vi "Measure.vi"(8 "error in (no error)":errorcluster, 11 "Measurement2D in":refnum<class "Measurement2D.lvclass">) -> (0 "error out":errorcluster, 1 "Current Value":dbl, 2 "Result":dbl, 3 "Measurement2D out":refnum<class "Measurement2D.lvclass">)   [LabVIEW 2014, in "Measurement2D.lvclass"]
uses:
  Measurement2D.lvclass
  Instrument/Instrument/Instrument.lvclass
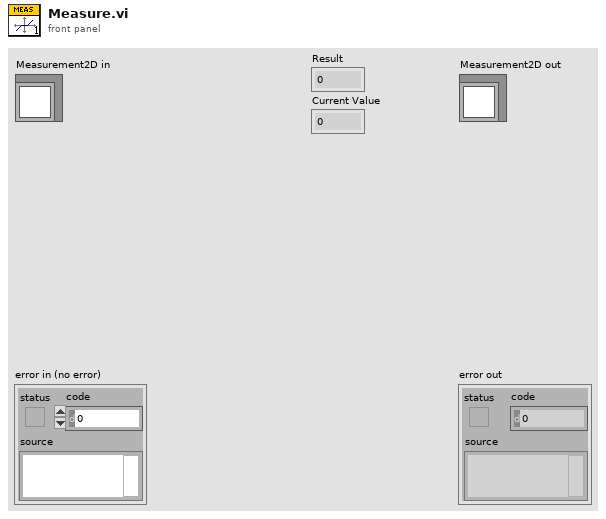
[diagram p1: front panel]
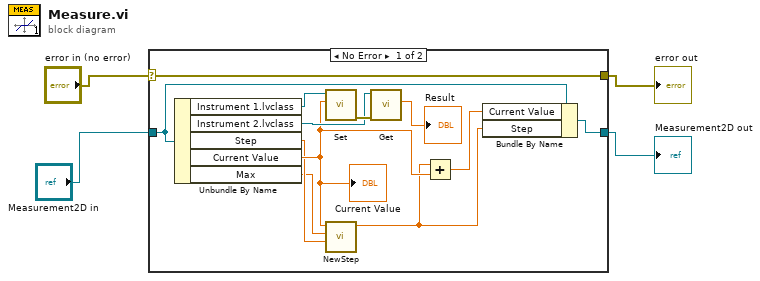
[diagram p0: block diagram]
diagram:
  n1 = case shown="No Error" "error in (no error)" {
    selector: "error in (no error)" -> [w16 w18]
    tunnel: [w16 w18] -> w3
    tunnel: [w13 w17] -> w1
    tunnel: "Measurement2D in" -> [w15 w17]
    frame No Error {
      n2 = Unbundle By Name(w15) -> ("Instrument 1.lvclass"=w12:refnum<class "Instrument.lvclass">, "Instrument 2.lvclass"=w9:refnum<class "Instrument.lvclass">, "Step"=w7:dbl, "Current Value"=w8:dbl, "Max"=w6:dbl)
      "Current Value" <- w8
      n3 = call-dynamic "Set.vi"("Numeric"=w8, "Instrument in"=w12) -> ("error out"=w11:errorcluster)  [unwired: 8 in, 1 out]
      n4 = call "NewStep.vi"("Step"=w7, "Max"=w6, "Current Value"=w8) -> ("Step 2"=w5:dbl)  [unwired: 8 in]
      n5 = call-dynamic "Get.vi"("error in (no error)"=w11, "Instrument in"=w9) -> ("Numeric"=→"Result":dbl)  [unwired: 7 in, 2 out]
      n6 = Add(x=w5, y=w8) -> (x+y=w14:dbl)
      n7 = Bundle By Name(cluster=w15, "Current Value"=w14, "Step"=w5) -> (w13:refnum<class "Measurement2D.lvclass">)
    }
    frame Error {
    }
  }
  "error out" <- w3
  "Measurement2D out" <- w1
